vi "Collide.vi"(9 "Team In":refnum<class "Team.lvclass">, 11 "MySquare in":refnum<class "MySquare.lvclass">) -> (1 "Team":refnum<class "Team.lvclass">, 3 "MySquare out":refnum<class "MySquare.lvclass">)   [LabVIEW 2020, in "The_Hill_Youth.lvlib" / "MySquare.lvclass"]
uses:
  MySquare.lvclass
  C:/dev/lv20CE/sol-squarebattle/ProjectTemplates/Source/SummerOfLabVIEW/SquareBattle/template/SquareBattle/Square/Square.lvclass
  SquareBattle/Team/Team.lvclass
  MyTeam/MyTeam.lvclass
  C:/dev/lv20CE/sol-squarebattle/ProjectTemplates/Source/SummerOfLabVIEW/SquareBattle/template/SquareBattle/Team/Team.lvclass
  MyTeam/map_point.ctl
  SquareBattle/Square/Square.lvclass/Square.ctl
  SquareBattle/Square/Square.lvclass
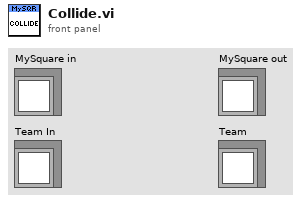
[diagram p1: front panel]
types:
  T1 = typedef "map_point.ctl" = cluster{"status":enum16{"unknown", "frind", "enemy", "empty"}, "plans":enum16{"stay", "duplicate", "attack", "move to", "no plans"}, "age":dbl}
  T2 = typedef "SquareBattle.lvlib/Position.ctl" = cluster{"Row":i32, "Col":i32}
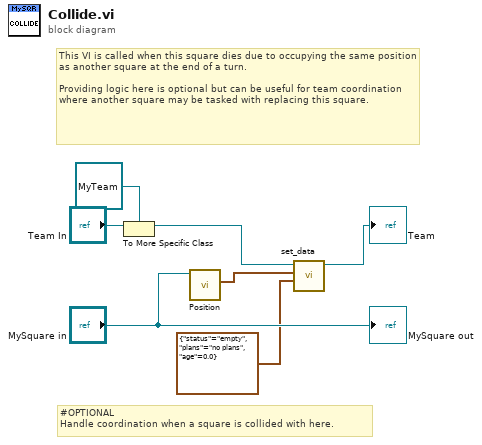
[diagram p0: block diagram]
diagram:
  # "#OPTIONAL\nHandle coordination when a square is collided with here."
  # "This VI is called when this square dies due to occupying the same position as another square at the end of a turn.\n\nProviding logic here is optional but can be useful for team coordination where another square may be tasked with replacing this square."
  n1 = To More Specific Class(target class=refnum<class "MyTeam.lvclass"> refnum ("SquareTeam.lvlib:MyTeam.lvclass"), reference="Team In") -> (specific class reference=w3:refnum<class "MyTeam.lvclass">)  [unwired: 1 in, 1 out]
  n2 = call "Position.vi"("Square in"="MySquare in") -> ("Position"=w4:T2)  [unwired: 10 in]
  n3 = call "set_data.vi"("new data"=T1 {"status"=enum."empty", "plans"=enum."no plans", "age"=0.0}, "point to set index"=w4, "SquareTeam.lvlib:MyTeam.lvclass 2"=w3) -> ("SquareTeam.lvlib:MyTeam.lvclass"=→"Team":refnum<class "MyTeam.lvclass">)  [unwired: 8 in]
  "MySquare out" <- "MySquare in"
